vi "Macros List to Item Names.vi"(0 "Macros List":cluster{"enabled?":bool, "macro name":string}[](array[cluster])) -> (1 "Item Names":string[][](array[string]), 2 "Array of Enabled?":bool[](array[boolean]))   [LabVIEW 2016, in "Hardware.lvlib" / "Motions.lvlib" / "Motions Configuration.lvclass"]
uses:
  <userlib>/Common Components/Hardware/Abstract System/Motions/Motions Config/Motions Configuration.lvclass
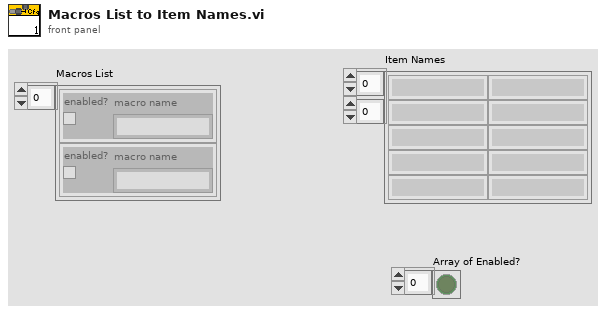
[diagram p1: front panel]
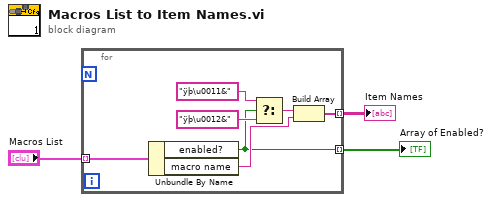
[diagram p0: block diagram]
diagram:
  n1 = for {
    tunnel: "Macros List" -> [w10] mode=indexing
    tunnel: [w5] -> w2 mode=indexing
    tunnel: [w4] -> w1 mode=indexing
    n2 = Unbundle By Name(w10) -> ("enabled?"=w4:bool, "macro name"=w6:string)
    n3 = Select(t="ÿþ\u0011&" ("string"), s=w4, f="ÿþ\u0012&") -> (s? t:f=w7:string)
    n4 = Build Array(w7, w6) -> (w5:string[])
  }
  "Item Names" <- w2
  "Array of Enabled?" <- w1
